vi "Get Column Widths.vi"(8 "error in (no error)":errorcluster, 11 "Multicolumn List Box View Model in":refnum<class "Multicolumn List Box View Model.lvclass">) -> (0 "error out":errorcluster, 2 "Widths":i32[](array[numeric]), 3 "Multicolumn List Box View Model out":refnum<class "Multicolumn List Box View Model.lvclass">)   [LabVIEW 2020, in "Multicolumn List Box View Model.lvclass"]
uses:
  Multicolumn List Box View Model.lvclass
  Multicolumn List Box View Model.lvclass/Multicolumn List Box View Model.ctl
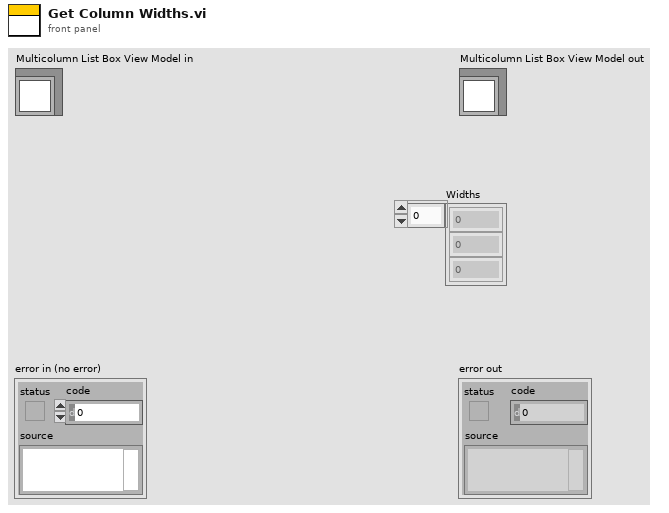
[diagram p1: front panel]
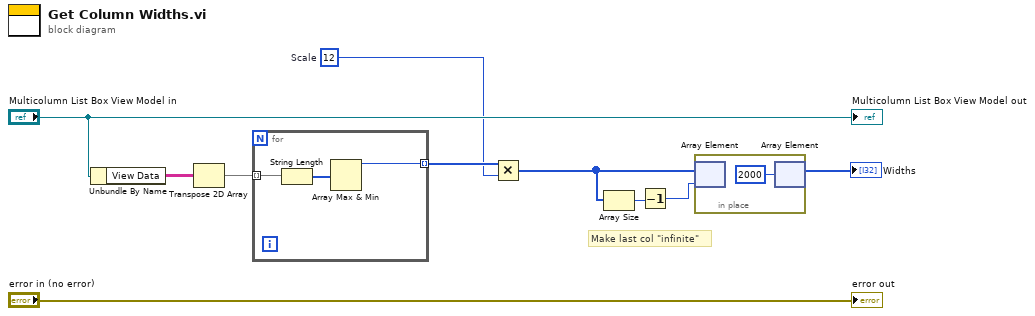
[diagram p0: block diagram]
diagram:
  w7 = 12  # Scale
  # "Make last col \"infinite\""
  n1 = Unbundle By Name("Multicolumn List Box View Model in") -> ("View Data"=w5:string[][])
  n2 = Transpose 2D Array(2D array=w5) -> (transposed array=w6:string[][])
  n3 = for {
    tunnel: w6 -> [w13] mode=indexing
    tunnel: [w11] -> w8 mode=indexing
    n4 = String Length(string=w13) -> (length=w12:i32[])
    n5 = Array Max & Min(array=w12) -> (max value=w11:i32)  [unwired: 3 out]
  }
  n6 = Multiply(x=w8, y=w7) -> (x*y=w3:i32[])
  n7 = Array Size(array=w3) -> (size(s)=w4:i32)
  n8 = Decrement(x=w4) -> (x-1=w1:i32)
  n9 = in-place {
    n10 = in-place-array #1(w3, w1) -> ()  [unwired: 1 out]
    n11 = in-place-array #1(2000 ("element")) -> (→"Widths":i32[])  [unwired: 1 out]
  }
  "error out" <- "error in (no error)"
  "Multicolumn List Box View Model out" <- "Multicolumn List Box View Model in"
